vi "WriteStringData.vi"(8 "Error In":errorcluster caption="エラー入力", 9 "文字列":string, 10 "データ":cluster{"セクション":string, "キー":string}, 11 "refnum":T1) -> (0 "Error Out":errorcluster caption="エラー出力", 3 "refnum out":T1 caption="refnum出力")   [LabVIEW 2015]
doc: "iniファイルから文字列データを読み込みます。"
uses:
  <vilib>/Utility/config.llb/Config Data RefNum.ctl
  <vilib>/Utility/config.llb/Write Key (String).vi
  <vilib>/Utility/config.llb/NI_LVConfig.lvlib
panel:
  # "■Iniファイルへ文字列データを書き込む"
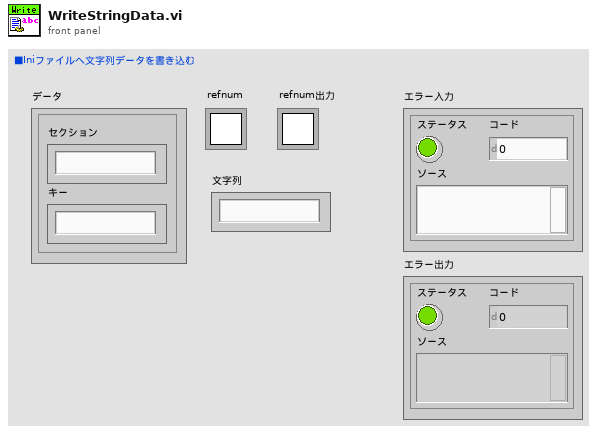
[diagram p1: front panel]
types:
  T1 = typedef "NI_LVConfig.lvlib/Config Data RefNum.ctl" = refnum<k1>
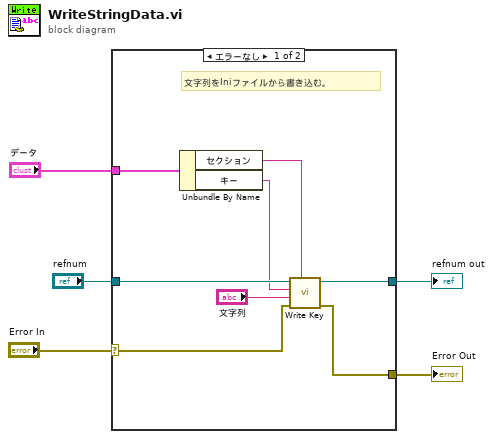
[diagram p0: block diagram]
diagram:
  n1 = case shown="エラーなし" "Error In" {
    selector: "Error In" -> [w9 w15]
    tunnel: [w6 w15] -> w5
    tunnel: "データ" -> [w13 _]
    tunnel: [w7 w14] -> w2
    tunnel: "refnum" -> [w12 w14]
    frame No Error {
      # "文字列をIniファイルから書き込む。"
      n2 = Unbundle By Name(w13) -> ("セクション"=w11:string, "キー"=w10:string)
      n3 = call-poly <vilib>:"Write Key.vi"("section"=w11, "error in (no error)"=w9, "value"="文字列", "key"=w10, "refnum"=w12) -> ("error out"=w6:errorcluster, "refnum out"=w7:T1)  [unwired: 4 in, 1 out]
    }
    frame Error {
    }
  }
  "Error Out" <- w5
  "refnum out" <- w2
